vi "getName.vi"(0 "reference":refnum<class "ActorNode.lvclass">, 5 "error in (no error)":errorcluster) -> (14 "reference out":refnum<class "ActorNode.lvclass">, 15 "name":refnum<class "MultiLineString.lvclass">, 19 "error out":errorcluster)   [LabVIEW 2014, in "ActorNode.lvclass"]
doc: "public MultiLineString getName()"
uses:
  <resource>/Framework/Providers/Open_GDS/UML/ActorNode_class/ActorNode.lvclass
  <resource>/Framework/Providers/Open_GDS/UML/MultiLineString_class/MultiLineString.lvclass
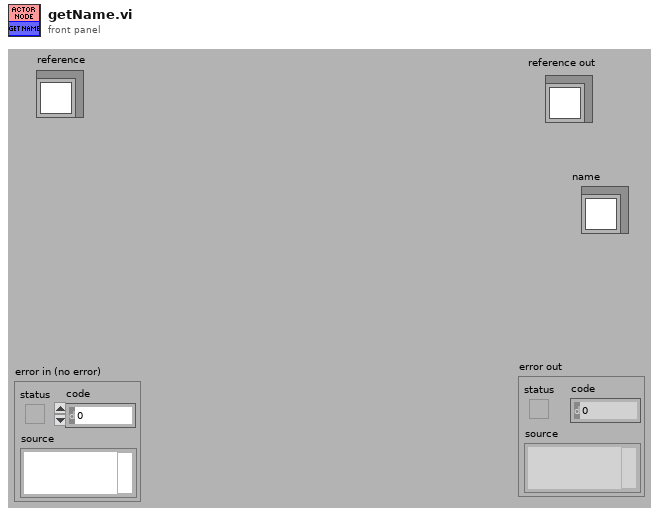
[diagram p1: front panel]
types:
  T1 = typedef "ActorNode.lvclass/ObjectAttributes.ctl" = cluster{"name":refnum<class "MultiLineString.lvclass">, "DEFAULT_WIDTH":i32, "DEFAULT_HEIGHT":i32, "DEFAULT_GAP":i32}
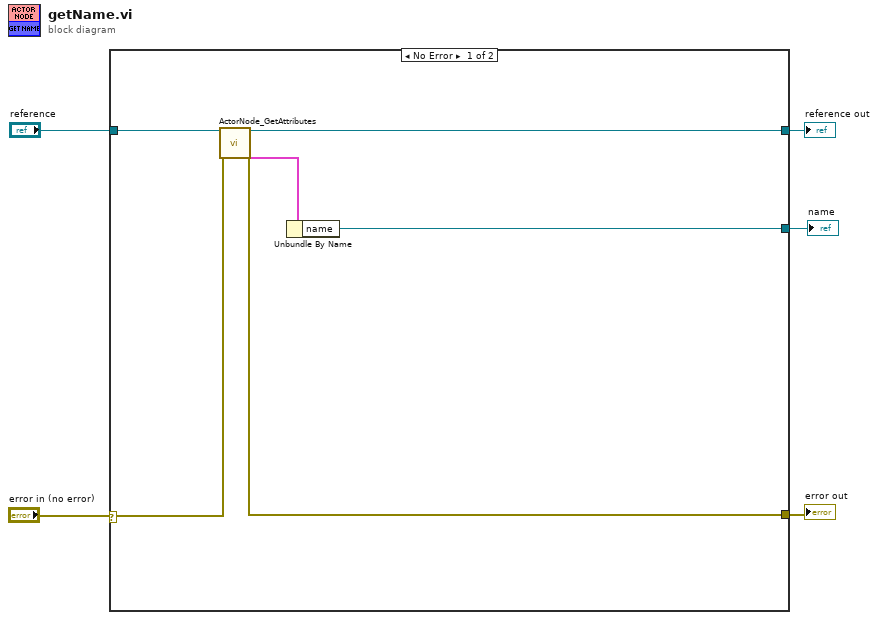
[diagram p0: block diagram]
diagram:
  n1 = case shown="No Error" "error in (no error)" {
    selector: "error in (no error)" -> [w8 w12]
    tunnel: "reference" -> [w11 w13]
    tunnel: [w10 w12] -> w4
    tunnel: [w9 w13] -> w3
    tunnel: [w7 _] -> w1
    frame No Error {
      n2 = call <resource>:"ActorNode_GetAttributes.vi"("reference in"=w11, "error in (no error)"=w8) -> ("reference out"=w9:refnum<class "ActorNode.lvclass">, "Data"=w6:T1, "error out"=w10:errorcluster)  [unwired: 1 in, 14 out]
      n3 = Unbundle By Name(w6) -> ("name"=w7:refnum<class "MultiLineString.lvclass">)
    }
    frame Error {
    }
  }
  "reference out" <- w3
  "error out" <- w4
  "name" <- w1
